vi "Save NI to Configuration File.vi"(5 "NI1":dbl, 7 "NI2":dbl) -> ()   [LabVIEW 2017]
uses:
  <vilib>/Utility/config.llb/Write Key (Double).vi
  <vilib>/Utility/config.llb/NI_LVConfig.lvlib
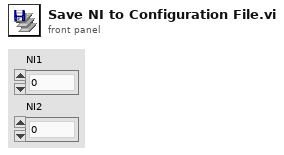
[diagram p1: front panel]
types:
  T1 = typedef "NI_LVConfig.lvlib/Config Data RefNum.ctl" = refnum<k1>
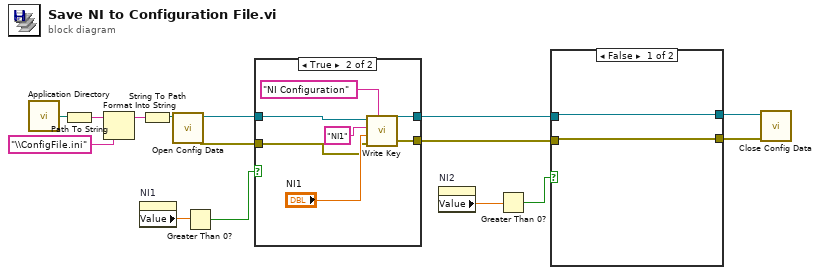
[diagram p0: block diagram]
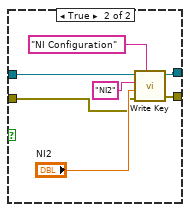
[diagram p2: hidden frame]
diagram:
  n1 = call <vilib>:"Application Directory.vi"() -> ("Application Directory"=w15:path)
  n2 = Path To String(path=w15) -> (string=w14:string)
  n3 = Format Into String(initial string=w14, "\\ConfigFile.ini" ("string")) -> (resulting string=w12:string)  [unwired: 2 in, 1 out]
  n4 = property on="NI1" class="DigNum (strict)"() -> ("Value"=w4:dbl)  [unwired: 2 in, 2 out]
  n5 = String To Path(string=w12) -> (path=w11:path)
  n6 = call <vilib>:"Open Config Data.vi"("configuration file path"=w11) -> ("error out"=w5:errorcluster, "refnum"=w10:T1)  [unwired: 8 in, 1 out]
  n7 = Greater Than 0?(x=w4) -> (x > 0?=w3:bool)
  n8 = case shown="True" w3 {
    tunnel: w10 -> [w17 w24]
    tunnel: [w17 w21] -> w9
    tunnel: [w16 w19] -> w6
    tunnel: w5 -> [w16 w18]
    frame False {
    }
    frame True {
      n9 = call-poly <vilib>:"Write Key.vi"("section"="NI Configuration", "error in (no error)"=w18, "value"="NI1", "key"="NI1", "refnum"=w24) -> ("error out"=w19:errorcluster, "refnum out"=w21:T1)  [unwired: 4 in, 1 out]
    }
  }
  n10 = property on="NI2" class="DigNum (strict)"() -> ("Value"=w2:dbl)  [unwired: 2 in, 2 out]
  n11 = Greater Than 0?(x=w2) -> (x > 0?=w1:bool)
  n12 = case shown="False" w1 {
    tunnel: w9 -> [w26 w31]
    tunnel: [w26 w29] -> w8
    tunnel: [w25 w28] -> w7
    tunnel: w6 -> [w25 w27]
    frame False {
    }
    frame True {
      n13 = call-poly <vilib>:"Write Key.vi"("section"="NI Configuration", "error in (no error)"=w27, "value"="NI2", "key"="NI2", "refnum"=w31) -> ("error out"=w28:errorcluster, "refnum out"=w29:T1)  [unwired: 4 in, 1 out]
    }
  }
  n14 = call <vilib>:"Close Config Data.vi"("error in (no error)"=w7, "refnum"=w8) -> ()  [unwired: 8 in, 2 out]
